vi "Buffer.Double.vi"(8 "error in (no error)":errorcluster, 10 "buffer in":dbl[](array[numeric]), 11 "buffer size":i32) -> (0 "error out":errorcluster, 2 "buffer out":dbl[](array[numeric]))   [LabVIEW 2016, in "VeriStand Data.lvlib"]
uses:
  VeriStand Data.lvlib
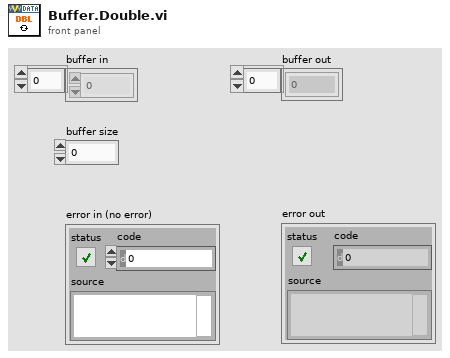
[diagram p1: front panel]
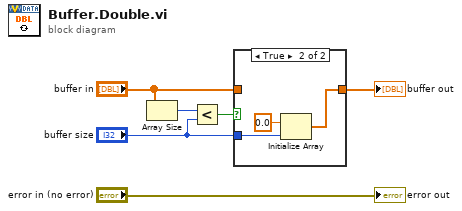
[diagram p0: block diagram]
diagram:
  n1 = Array Size(array="buffer in") -> (size(s)=w5:i32)
  n2 = Less?(x=w5, y="buffer size") -> (x < y?=w3:bool)
  n3 = case shown="True" w3 {
    tunnel: "buffer in" -> [w7 _]
    tunnel: "buffer size" -> [_ w9]
    tunnel: [w7 w8] -> w2
    frame False {
    }
    frame True {
      n4 = Initialize Array(0.0 ("element"), w9) -> (w8:dbl[])
    }
  }
  "buffer out" <- w2
  "error out" <- "error in (no error)"
